vi "convert mass and density to liters.vi"(7 "Density unit (str)":string, 10 "Density":dbl, 11 "Mass total in (kg)":dbl) -> (2 "Volume out (l)":dbl)   [LabVIEW 2013]
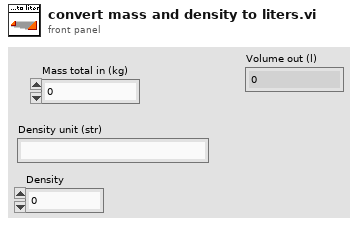
[diagram p1: front panel]
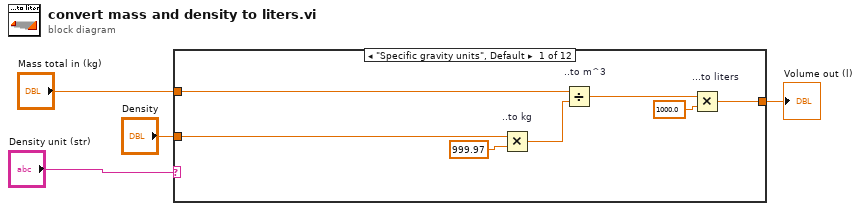
[diagram p0: block diagram]
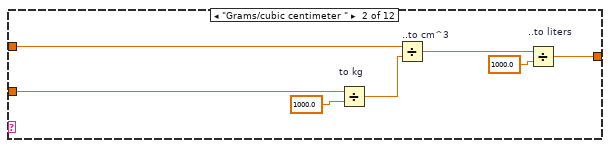
[diagram p2: hidden frame]
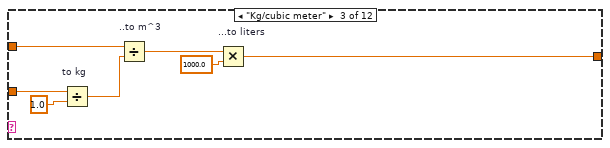
[diagram p3: hidden frame]
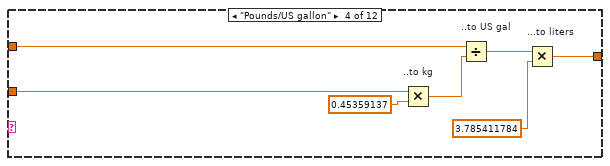
[diagram p4: hidden frame]
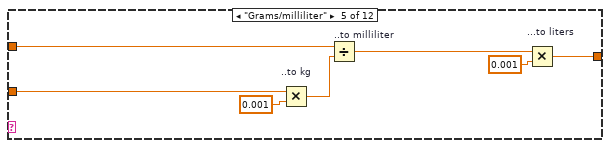
[diagram p5: hidden frame]
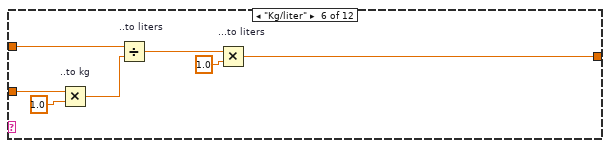
[diagram p6: hidden frame]
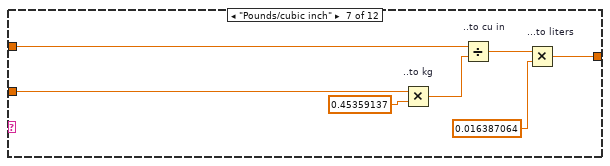
[diagram p7: hidden frame]
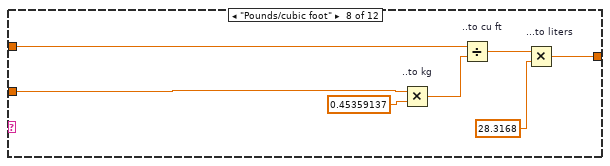
[diagram p8: hidden frame]
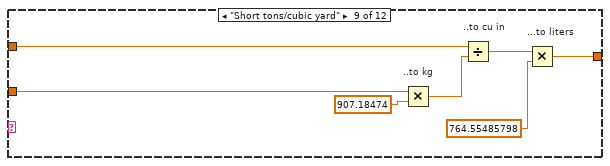
[diagram p9: hidden frame]
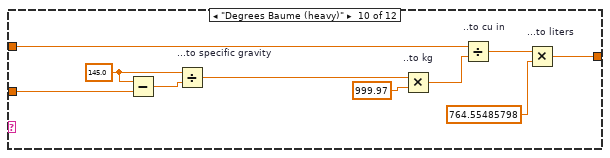
[diagram p10: hidden frame]
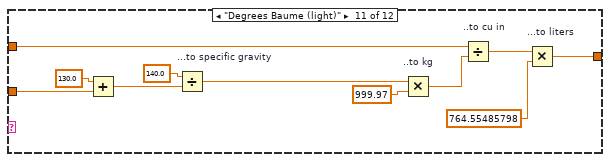
[diagram p11: hidden frame]
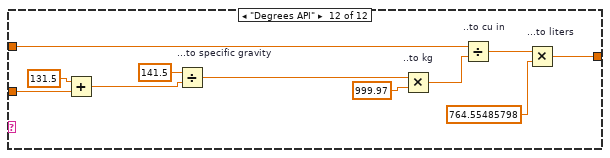
[diagram p12: hidden frame]
diagram:
  n1 = case shown="\"Specific gravity units\", Default" "Density unit (str)" {
    tunnel: "Mass total in (kg)" -> [w6 w15 w22 w29 w36 w43 w51 w56 w65 w76 w87 w98]
    tunnel: "Density" -> [w7 w18 w25 w32 w39 w46 w53 w54 w67 w71 w82 w93]
    tunnel: [w5 w12 w19 w26 w33 w40 w48 w55 w62 w73 w84 w95] -> w2
    frame "Specific gravity units", Default {
      n2 = Multiply "..to kg"(x=w7, y=999.97) -> (x*y=w11:dbl)
      n3 = Divide "..to m^3"(x=w6, y=w11) -> (x/y=w10:dbl)
      n4 = Multiply "...to liters"(x=w10, y=1000.0) -> (x*y=w5:dbl)
    }
    frame "Grams/cubic centimeter " {
      n5 = Divide "to kg"(x=w18, y=1000.0) -> (x/y=w16:dbl)
      n6 = Divide "..to cm^3"(x=w15, y=w16) -> (x/y=w14:dbl)
      n7 = Divide "..to liters"(x=w14, y=1000.0) -> (x/y=w12:dbl)
    }
    frame "Kg/cubic meter" {
      n8 = Divide "to kg"(x=w25, y=1.0) -> (x/y=w23:dbl)
      n9 = Divide "..to m^3"(x=w22, y=w23) -> (x/y=w21:dbl)
      n10 = Multiply "...to liters"(x=w21, y=1000.0) -> (x*y=w19:dbl)
    }
    frame "Pounds/US gallon" {
      n11 = Multiply "..to kg"(x=w32, y=0.45359137) -> (x*y=w30:dbl)
      n12 = Divide "..to US gal"(x=w29, y=w30) -> (x/y=w28:dbl)
      n13 = Multiply "...to liters"(x=w28, y=3.785411784) -> (x*y=w26:dbl)
    }
    frame "Grams/milliliter" {
      n14 = Multiply "..to kg"(x=w39, y=0.001) -> (x*y=w37:dbl)
      n15 = Divide "..to milliliter"(x=w36, y=w37) -> (x/y=w35:dbl)
      n16 = Multiply "...to liters"(x=w35, y=0.001) -> (x*y=w33:dbl)
    }
    frame "Kg/liter" {
      n17 = Multiply "..to kg"(x=w46, y=1.0) -> (x*y=w44:dbl)
      n18 = Divide "..to liters"(x=w43, y=w44) -> (x/y=w42:dbl)
      n19 = Multiply "...to liters"(x=w42, y=1.0) -> (x*y=w40:dbl)
    }
    frame "Pounds/cubic inch" {
      n20 = Multiply "..to kg"(x=w53, y=0.45359137) -> (x*y=w52:dbl)
      n21 = Divide "..to cu in"(x=w51, y=w52) -> (x/y=w50:dbl)
      n22 = Multiply "...to liters"(x=w50, y=0.016387064) -> (x*y=w48:dbl)
    }
    frame "Pounds/cubic foot" {
      n23 = Multiply "..to kg"(x=w54, y=0.45359137) -> (x*y=w60:dbl)
      n24 = Divide "..to cu ft"(x=w56, y=w60) -> (x/y=w59:dbl)
      n25 = Multiply "...to liters"(x=w59, y=28.3168) -> (x*y=w55:dbl)
    }
    frame "Short tons/cubic yard" {
      n26 = Multiply "..to kg"(x=w67, y=907.18474) -> (x*y=w66:dbl)
      n27 = Divide "..to cu in"(x=w65, y=w66) -> (x/y=w64:dbl)
      n28 = Multiply "...to liters"(x=w64, y=764.55485798) -> (x*y=w62:dbl)
    }
    frame "Degrees Baume (heavy)" {
      w69 = 145.0 ("y")
      n29 = Subtract(x=w69, y=w71) -> (x-y=w70:dbl)
      n30 = Divide "...to specific gravity"(x=w69, y=w70) -> (x/y=w68:dbl)
      n31 = Multiply "..to kg"(x=w68, y=999.97) -> (x*y=w77:dbl)
      n32 = Divide "..to cu in"(x=w76, y=w77) -> (x/y=w75:dbl)
      n33 = Multiply "...to liters"(x=w75, y=764.55485798) -> (x*y=w73:dbl)
    }
    frame "Degrees Baume (light)" {
      n34 = Add(x=130.0 ("y"), y=w82) -> (x+y=w81:dbl)
      n35 = Divide "...to specific gravity"(x=140.0 ("y"), y=w81) -> (x/y=w79:dbl)
      n36 = Multiply "..to kg"(x=w79, y=999.97) -> (x*y=w88:dbl)
      n37 = Divide "..to cu in"(x=w87, y=w88) -> (x/y=w86:dbl)
      n38 = Multiply "...to liters"(x=w86, y=764.55485798) -> (x*y=w84:dbl)
    }
    frame "Degrees API" {
      n39 = Add(x=131.5 ("y"), y=w93) -> (x+y=w92:dbl)
      n40 = Divide "...to specific gravity"(x=141.5 ("y"), y=w92) -> (x/y=w90:dbl)
      n41 = Multiply "..to kg"(x=w90, y=999.97) -> (x*y=w99:dbl)
      n42 = Divide "..to cu in"(x=w98, y=w99) -> (x/y=w97:dbl)
      n43 = Multiply "...to liters"(x=w97, y=764.55485798) -> (x*y=w95:dbl)
    }
  }
  "Volume out (l)" <- w2
